vi "Read Deadband.vi"(8 "error in (no error)":cluster{"状态":bool, "代码":i32, "源":string} caption="错误输入（无错误）", 11 "水位控制器输入":refnum<class "Level Controller.lvclass">) -> (0 "error out":cluster{"状态":bool, "代码":i32, "源":string} caption="错误输出", 2 "死区":T1, 3 "水位控制器输出":refnum<class "Level Controller.lvclass">)   [LabVIEW 2013, in "Level Controller.lvlib" / "Level Controller.lvclass"]
doc: "读取水位控制器的死区范围。"
uses:
  Level Controller.lvclass
  Deadband.ctl
  Level Controller.lvclass/Level Controller.ctl
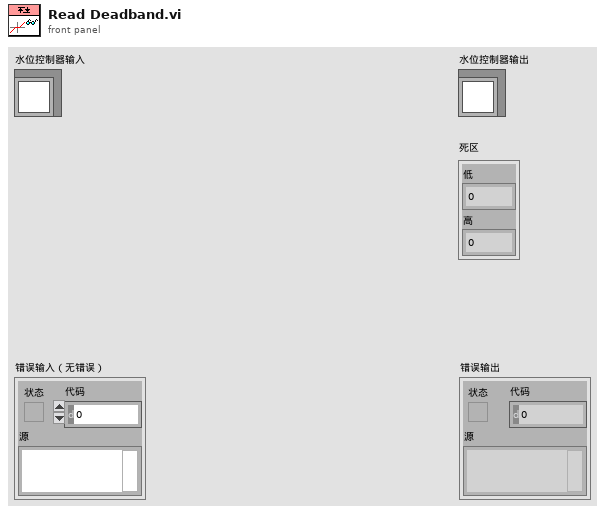
[diagram p1: front panel]
types:
  T1 = typedef "Level Controller.lvlib/Level Controller.lvclass/Deadband.ctl" = cluster{"Low":dbl, "High":dbl}
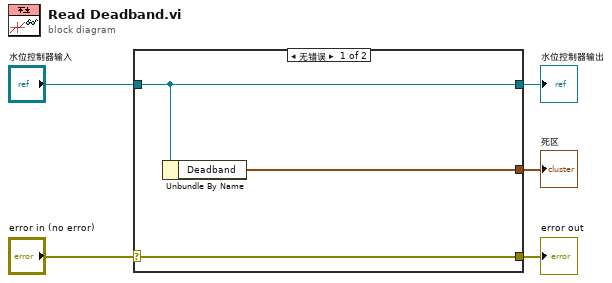
[diagram p0: block diagram]
diagram:
  n1 = case shown="无错误" "error in (no error)" {
    selector: "error in (no error)" -> [w8 w9]
    tunnel: [w8 w9] -> w4
    tunnel: [w7 w10] -> w3
    tunnel: "水位控制器输入" -> [w7 w10]
    tunnel: [w6 _] -> w2
    frame No Error {
      n2 = Unbundle By Name(w7) -> ("Deadband"=w6:T1)
    }
    frame Error {
    }
  }
  "error out" <- w4
  "水位控制器输出" <- w3
  "死区" <- w2
